vi "Keithley2200series.vi"() -> ()   [LabVIEW 2014]
uses:
  <vilib>/Utility/file.llb/Write To Spreadsheet File (string).vi
  C:/Users/rad/Desktop/Keithley 2200 Series Power Supplies Ver 1.2 (LV2009)/Keithley 2200 Series/Keithley 2200 Series.lvlib
panel:
  in  "Файл записи замеров":path
  in  "OCP, A":dbl format="%.2f"
  out "error out":errorcluster
  out "Ток, А":string
  in  "VISA resource name":refnum<visa-resource-name>
  in  "stop":bool
  in  "Напряжение, В":dbl
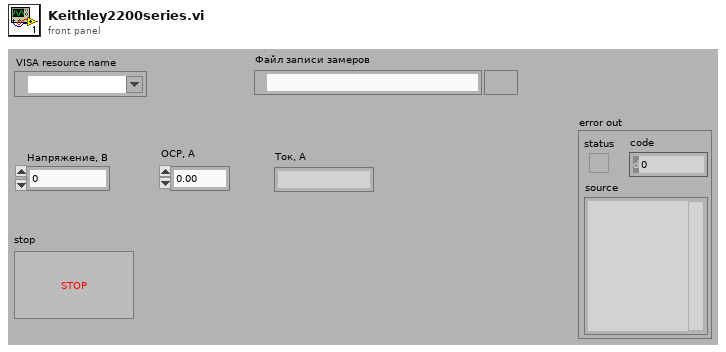
[diagram p1: front panel]
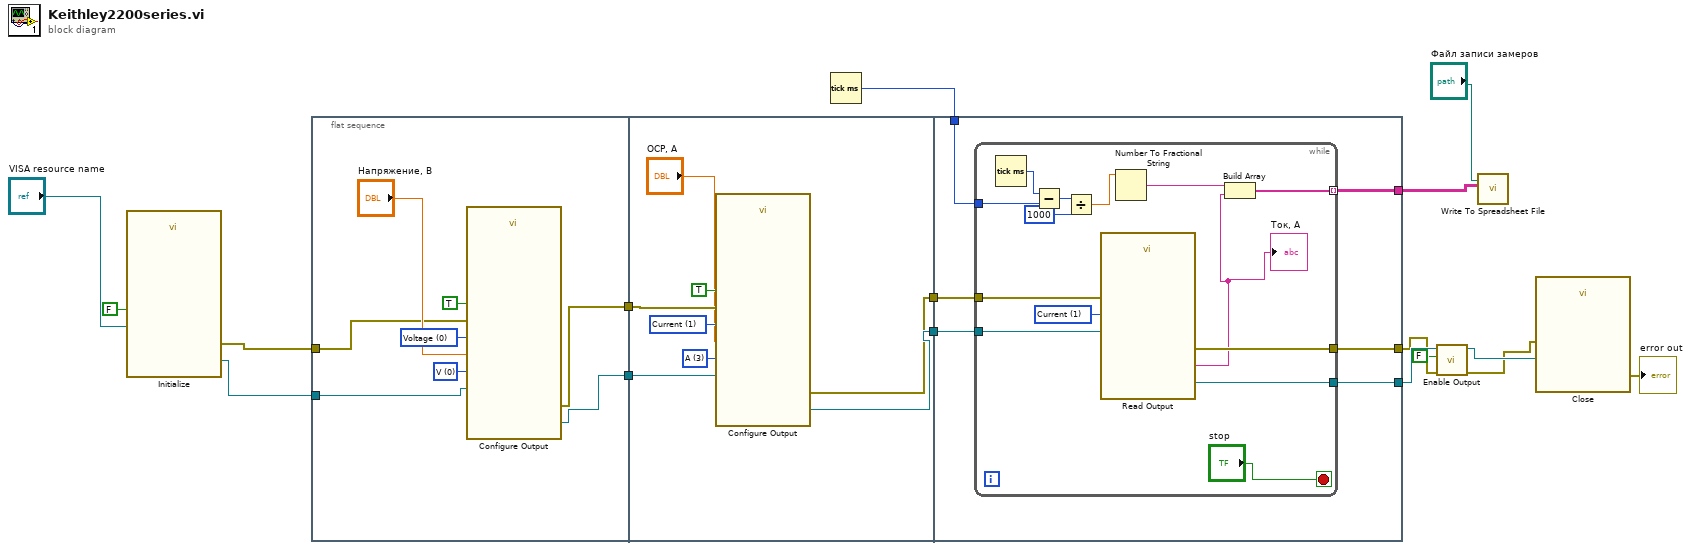
[diagram p0: block diagram]
diagram:
  n1 = call "Initialize.vi"("Reset (True)"=FALSE, "VISA resource name"="VISA resource name") -> ("error out"=w14:errorcluster, "VISA resource name out"=w15:refnum<visa-resource-name>)  [unwired: 8 in]
  n2 = flat-sequence {
    tunnel: w15 -> [w23]
    tunnel: w14 -> [w22]
    tunnel: [w21] -> w12
    tunnel: [w20] -> w10
    tunnel: w12 -> [w31]
    tunnel: [w27] -> w11
    tunnel: w10 -> [w32]
    tunnel: [w26] -> w9
    tunnel: w11 -> [w39]
    tunnel: w9 -> [w38]
    tunnel: [w37] -> w4
    tunnel: [w36] -> w5
    tunnel: w8 -> [w35]
    tunnel: [w34] -> w7
    frame #0 {
      w18 = u16 0 items=["Voltage", "Current"] ("Function(0:Voltage)")
      w19 = u16 0 items=["V", "mV", "kV", "A", "mA"] ("Unit(V)")
      n3 = call "Configure Output.vi"("VISA resource name"=w23, "Manual Range(0.00)"="Напряжение, В", "Function(0:Voltage)"=w18, "Enable Output (T: Enable)"=TRUE, "error in (no error)"=w22, "Unit(V)"=w19) -> ("VISA resource name out"=w21:refnum<visa-resource-name>, "error out"=w20:errorcluster)  [unwired: 8 in]
    }
    frame #1 {
      w29 = u16 3 items=["V", "mV", "kV", "A", "mA"] ("Unit(V)")
      w30 = u16 1 items=["Voltage", "Current"] ("Function(0:Voltage)")
      n4 = call "Configure Output.vi"("VISA resource name"=w31, "Manual Range(0.00)"="OCP, A", "Function(0:Voltage)"=w30, "Enable Output (T: Enable)"=TRUE, "error in (no error)"=w32, "Unit(V)"=w29) -> ("VISA resource name out"=w27:refnum<visa-resource-name>, "error out"=w26:errorcluster)  [unwired: 8 in]
    }
    frame #2 {
      n5 = while {
        tunnel: w39 -> [w52]
        tunnel: w38 -> [w51]
        tunnel: [w50] -> w37
        tunnel: [w49] -> w36
        tunnel: w35 -> [w46]
        tunnel: [w43] -> w34 mode=indexing
        stop <- "stop" stop-if-true
        w48 = u16 1 items=["Voltage", "Current", "Power"] ("Measurement Function (0:Voltage)")
        n6 = Tick Count (ms)() -> (millisecond timer value=w47:u32)
        n7 = Subtract(x=w47, y=w46) -> (x-y=w42:u32)
        n8 = Divide(x=w42, y=u32 1000) -> (x/y=w40:dbl)
        n9 = call "Read Output.vi"("VISA resource name"=w52, "Measurement Function (0:Voltage)"=w48, "error in (no error)"=w51) -> ("VISA resource name out"=w49:refnum<visa-resource-name>, "Measurement"=w45:string, "error out"=w50:errorcluster)  [unwired: 10 in]
        "Ток, А" <- w45
        n10 = Number To Fractional String(number=w40) -> (F-format string=w44:string)  [unwired: 3 in]
        n11 = Build Array(w44, w45) -> (w43:string[])
      }
    }
  }
  n12 = Tick Count (ms)() -> (millisecond timer value=w8:u32)
  n13 = call "Enable Output.vi"("error in (no error)"=w4, "Enable Output (T: Enable)"=FALSE, "VISA resource name"=w5) -> ("error out"=w1:errorcluster, "VISA resource name out"=w2:refnum<visa-resource-name>)  [unwired: 7 in]
  n14 = call-poly <vilib>:"Write To Spreadsheet File.vi"("2D data"=w7, "file path (dialog if empty)"="Файл записи замеров") -> ()  [unwired: 6 in, 1 out]
  n15 = call "Close.vi"("error in (no error)"=w1, "VISA resource name"=w2) -> ("error out"=→"error out":errorcluster)  [unwired: 9 in]
